vi "Change Epsilon.vi"(10 "new epsilon":dbl, 11 "AD* in":refnum<class "NI_Robotics_AnytimeDStar.lvclass">) -> (3 "AD* out":refnum<class "NI_Robotics_AnytimeDStar.lvclass">)   [LabVIEW 2017, in "NI_Robotics_AnytimeDStar.lvclass"]
uses:
  <vilib>/robotics/Navigation/Anytime D Star/NI_Robotics_AnytimeDStar.lvclass
  <vilib>/robotics/Navigation/Anytime D Star/NI_Robotics_AnytimeDStar.lvclass/NI_Robotics_AnytimeDStar.ctl
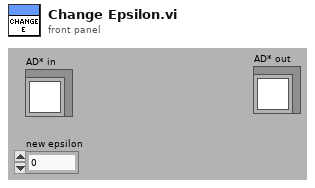
[diagram p1: front panel]
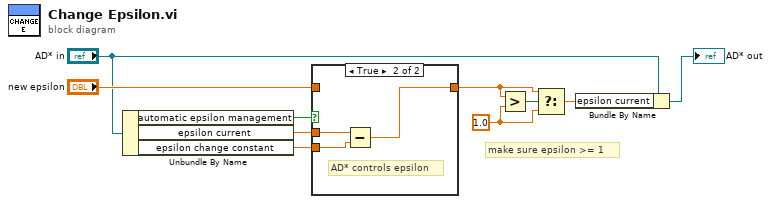
[diagram p0: block diagram]
diagram:
  w8 = 1.0 ("y")
  # "make sure epsilon >= 1"
  n1 = Unbundle By Name("AD* in") -> ("automatic epsilon management"=w6:bool, "epsilon current"=w5:dbl, "epsilon change constant"=w3:dbl)
  n2 = case shown="True" w6 {
    tunnel: [w11 w12] -> w7
    tunnel: w5 -> [_ w13]
    tunnel: "new epsilon" -> [w11 _]
    tunnel: w3 -> [_ w14]
    frame False {
    }
    frame True {
      # "AD* controls epsilon"
      n3 = Subtract(x=w13, y=w14) -> (x-y=w12:dbl)
    }
  }
  n4 = Greater?(x=w7, y=w8) -> (0:w9:bool)
  n5 = Select(t=w7, s=w9, f=w8) -> (s? t:f=w2:dbl)
  n6 = Bundle By Name(cluster="AD* in", "epsilon current"=w2) -> (→"AD* out":refnum<class "NI_Robotics_AnytimeDStar.lvclass">)
